vi "Timer_CalcDropSpeed.vi"(2 "LinesCleared":u8) -> (16 "DropSpeed(ms)":u16)   [LabVIEW 2018]
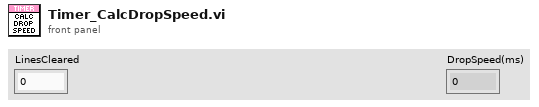
[diagram p1: front panel]
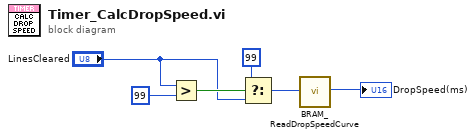
[diagram p0: block diagram]
diagram:
  n1 = Greater?(x="LinesCleared", y=u8 99) -> (0:w4:bool)
  n2 = Select(t=u8 99, s=w4, f="LinesCleared") -> (s? t:f=w2:u8)
  n3 = call "BRAM_ReadDropSpeedCurve.vi"("Address"=w2) -> ("DropSpeed(ms)"=→"DropSpeed(ms)":u16)  [unwired: 18 in]
